vi "Save_protocol.vi"(1 "Protocol cluster":T1={"Sequence"=["SIMPLE 2A+", "SIMPLE 1A+"], "Rel. requency"=[1.0, 1.0], "Frequency"=[0.5, 0.5], "Sequence interval"=200.0, "Rarest sequence "=200.0, "Randomization"=2} {"Randomization" items=["None", "Simple shuffle", "Block"]}, 2 "Protocol File Path":path) -> ()   [LabVIEW 2016]
uses:
  <vilib>/Utility/xml.llb/Write to XML File(string).vi
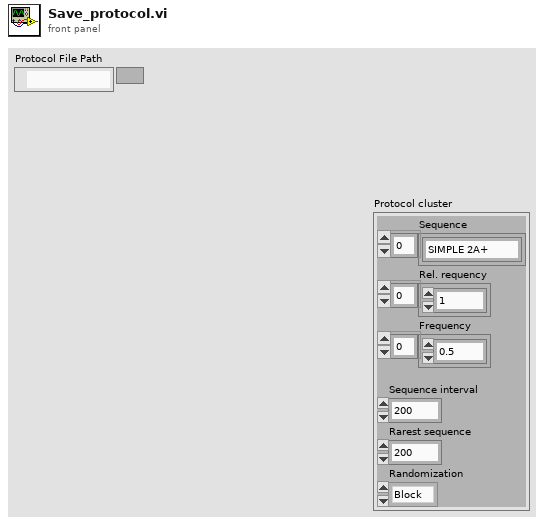
[diagram p1: front panel]
types:
  T1 = cluster{"Sequence":string[], "Rel. requency":dbl[], "Frequency":dbl[], "Sequence interval":dbl, "Rarest sequence ":dbl, "Randomization":u16}
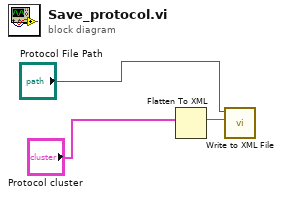
[diagram p0: block diagram]
diagram:
  n1 = Flatten To XML(anything="Protocol cluster") -> (xml string=w3:string)
  n2 = call-poly <vilib>:"Write to XML File.vi"("XML Input"=w3, "XML File Path"="Protocol File Path") -> ()  [unwired: 7 in, 3 out]
